vi "PS PassWord.vi"(1 "OK Button":bool, 2 "Password":string) -> (0 "Password Correct":bool)   [LabVIEW 2020]
panel:
  # "Enter Password and hit OK"
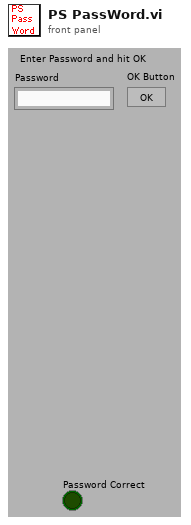
[diagram p1: front panel]
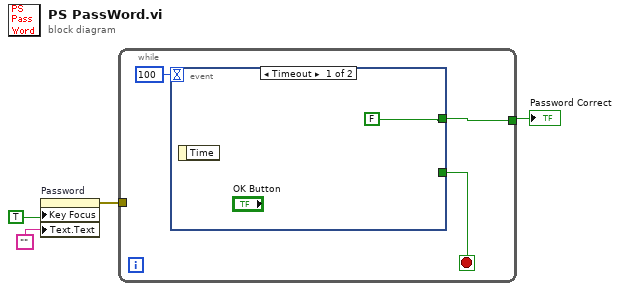
[diagram p0: block diagram]
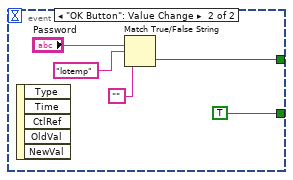
[diagram p2: hidden frame]
diagram:
  n1 = property on="Password" class="Str"("Key Focus"=TRUE, "Text.Text"="") -> (error out=w2:errorcluster)  [unwired: 2 in, 1 out]
  n2 = while {
    tunnel: [w6] -> w4
    tunnel: w2 -> [_]
    stop <- w5 stop-if-true
    n3 = event shown="[0] Timeout" {
      selector: _ -> [_ _]
      dyn-events: _ -> [_ _]
      timeout: 100 -> [_ _]
      tunnel: [FALSE w11] -> w6
      tunnel: [_ TRUE] -> w5
      event Timeout {
        n4 = event-data() -> ()  [unwired: 1 in, 1 out]
      }
      event "OK Button": Value Change {
        n5 = event-data() -> ()  [unwired: 1 in, 5 out]
        n6 = Match True/False String(2:"", 3:"lotemp" ("true string"), 4:"Password") -> (0:w11:bool)  [unwired: 1 out]
      }
    }
  }
  "Password Correct" <- w4
